vi "ReadFFLoop.vi"(0 "exptus":u32=20000, 1 "freq":u32, 2 "ExtTrig":u8, 3 "btrig_ch":u32, 4 "blocktrigger":u8) -> ()   [LabVIEW 2015]
uses:
  ESLSCDLL.dll
panel:
  # "lines for  FFTs, or 0 else"
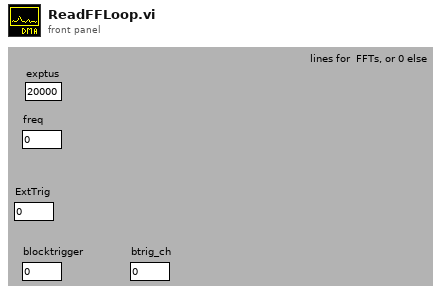
[diagram p1: front panel]
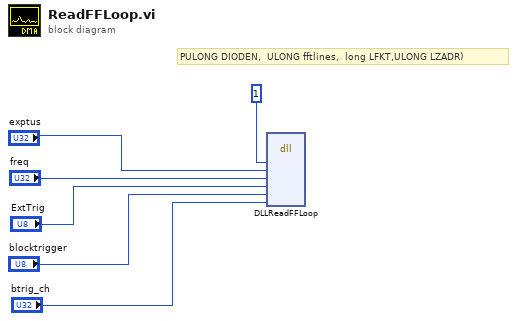
[diagram p0: block diagram]
diagram:
  # "PULONG DIODEN, \tULONG fftlines,  long LFKT,ULONG LZADR)"
  n1 = dll-call lib="C:/ENTW/PCIE/64bit/lv64/1cam/board.vis/ESLSCDLL.dll" fn="DLLReadFFLoop"("drv"=u32 1, "exptus"="exptus", "freq"="freq", "exttrig"="ExtTrig", "blocktrigger"="blocktrigger", "btrig_ch"="btrig_ch") -> ()  [unwired: 10 in, 2 out]
